vi "timeout.vi"(8 "error in (no error)":errorcluster, 11 "seconds to wait":dbl=0.2 min=0.2) -> (0 "error IO":errorcluster)   [LabVIEW 2017]
panel:
  out "Slide":u8(slide) scale=0.0..100.0
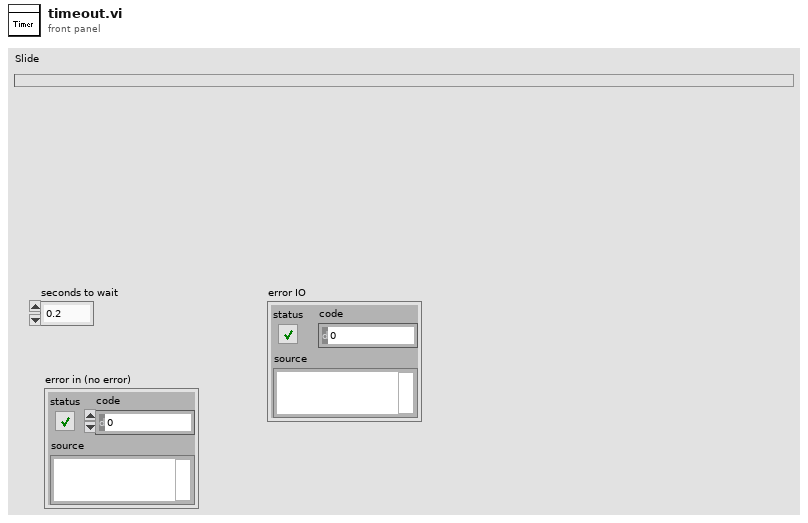
[diagram p1: front panel]
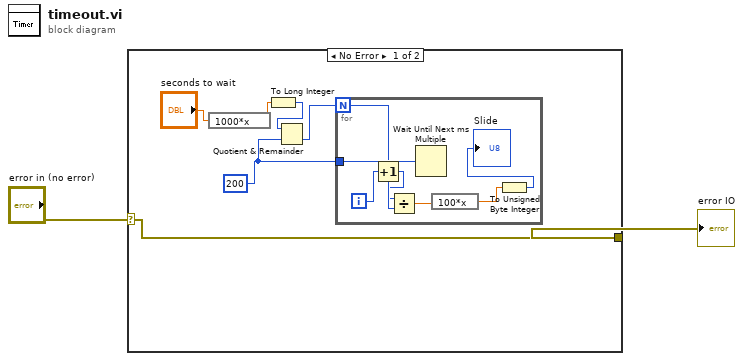
[diagram p0: block diagram]
diagram:
  n1 = case shown="No Error" "error in (no error)" {
    selector: "error in (no error)" -> [w8 w16]
    tunnel: [w8 w16] -> w1
    frame No Error {
      w4 = 200 ("millisecond multiple")
      n2 = expression code="1000*x"("seconds to wait") -> (w6:dbl)
      n3 = To Long Integer(number=w6) -> (32bit integer=w5:i32)
      n4 = Quotient & Remainder(x=w5, y=w4) -> (floor(x/y)=w3:i32)  [unwired: 1 out]
      n5 = for {
        N: w3 -> [w14]
        tunnel: w4 -> [w15]
        i -> [w10]
        n6 = Increment(x=w10) -> (x+1=w9:i32)
        n7 = Divide(x=w9, y=w14) -> (x/y=w13:dbl)
        n8 = Wait Until Next ms Multiple(millisecond multiple=w15) -> ()  [unwired: 1 out]
        n9 = expression code="100*x"(w13) -> (w12:dbl)
        n10 = To Unsigned Byte Integer(number=w12) -> (unsigned 8bit integer=→"Slide":u8)
      }
    }
    frame Error {
    }
  }
  "error IO" <- w1
